vi "Apply Z scale to XY.vi"(6 "Enlarge Z scale?":bool, 8 "error in (no error)":errorcluster, 10 "Z Axis Ref":refnum<vi>, 11 "Plot Area Ref":refnum<vi>) -> (0 "error out":errorcluster)   [LabVIEW 2017, in "2D Compass.lvclass"]
uses:
  <vilib>/Math Plots/2D Math Plots/2D Compass/2D Compass/2D Compass.lvclass
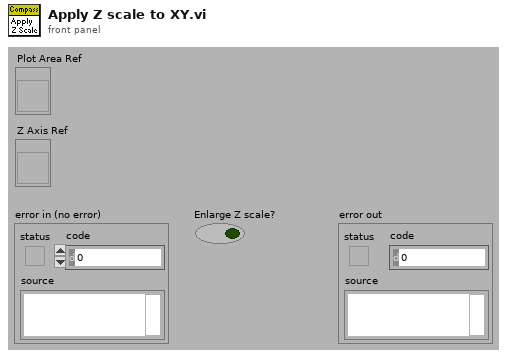
[diagram p1: front panel]
types:
  T1 = typedef "LVRectTypeDef.ctl" = cluster{"Left":i16, "Top":i16, "Right":i16, "Bottom":i16}
  T2 = typedef "LVPoint32TypeDef.ctl" = cluster{"Horizontal":i32, "Vertical":i32}
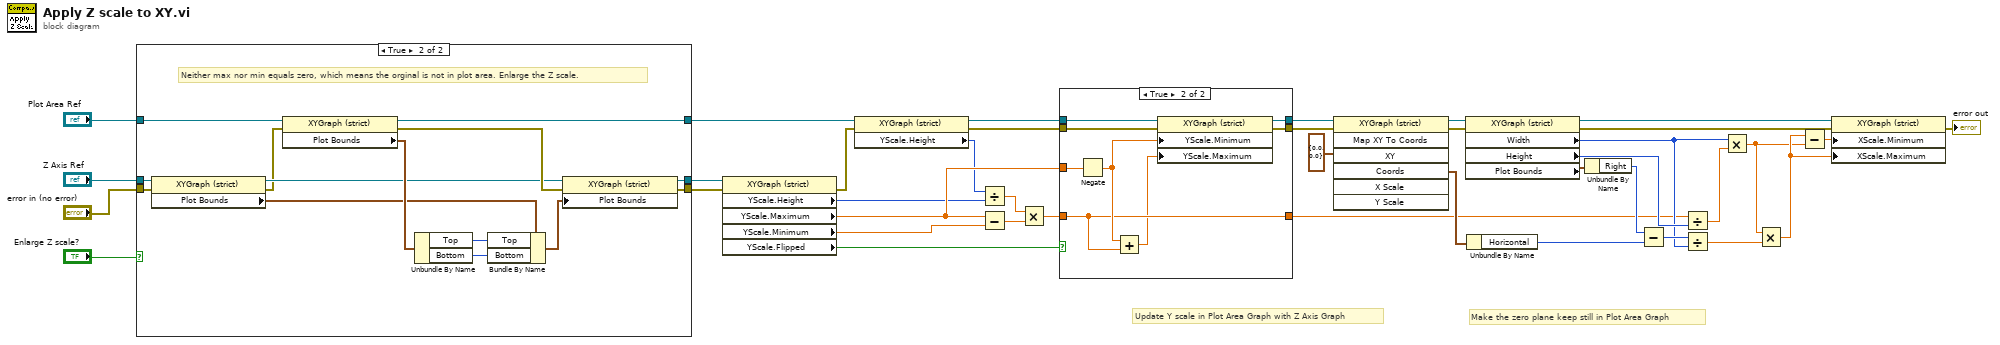
[diagram p0: block diagram]
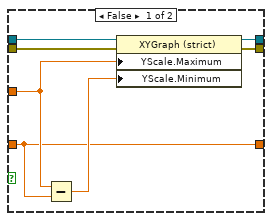
[diagram p3: hidden frame]
diagram:
  # "Make the zero plane keep still in Plot Area Graph"
  # "Update Y scale in Plot Area Graph with Z Axis Graph"
  n1 = case shown="True" "Enlarge Z scale?" {
    tunnel: [w40 w55] -> w6
    tunnel: "Plot Area Ref" -> [w40 w56]
    tunnel: [w42 w54] -> w4
    tunnel: "Z Axis Ref" -> [w42 w50]
    tunnel: [w41 w52] -> w2
    tunnel: "error in (no error)" -> [w41 w48]
    frame False {
    }
    frame True {
      # "Neither max nor min equals zero, which means the orginal is not in plot area. Enlarge the Z scale."
      n2 = property class="XYGraph (strict)"(reference=w50, error in=w48) -> (reference out=w49:refnum<vi>, error out=w47:errorcluster, "Plot Bounds"=w46:T1)
      n3 = property class="XYGraph (strict)"(reference=w56, error in=w47) -> (reference out=w55:refnum<vi>, error out=w53:errorcluster, "Plot Bounds"=w51:T1)
      n4 = Unbundle By Name(w51) -> ("Top"=w44:i16, "Bottom"=w43:i16)
      n5 = Bundle By Name(cluster=w46, "Top"=w44, "Bottom"=w43) -> (w45:T1)
      n6 = property class="XYGraph (strict)"(reference=w49, error in=w53, "Plot Bounds"=w45) -> (reference out=w54:refnum<vi>, error out=w52:errorcluster)
    }
  }
  n7 = property class="XYGraph (strict)"(reference=w4, error in=w2) -> (error out=w33:errorcluster, "YScale.Height"=w24:u32, "YScale.Maximum"=w32:dbl, "YScale.Minimum"=w31:dbl, "YScale.Flipped"=w30:bool)  [unwired: 1 out]
  n8 = property class="XYGraph (strict)"(reference=w6, error in=w33) -> (reference out=w26:refnum<vi>, error out=w34:errorcluster, "YScale.Height"=w25:u32)
  n9 = Divide(x=w25, y=w24) -> (x/y=w27:dbl)
  n10 = Subtract(x=w32, y=w31) -> (x-y=w28:dbl)
  n11 = Multiply(x=w27, y=w28) -> (x*y=w29:dbl)
  n12 = case shown="True" w30 {
    tunnel: w26 -> [w62 w70]
    tunnel: w29 -> [w58 w65]
    tunnel: w32 -> [w60 w67]
    tunnel: [w63 w71] -> w22
    tunnel: w34 -> [w61 w69]
    tunnel: [w58 w65] -> w9
    tunnel: [w57 w68] -> w23
    frame False {
      n13 = Subtract(x=w60, y=w58) -> (x-y=w59:dbl)
      n14 = property class="XYGraph (strict)"(reference=w62, error in=w61, "YScale.Maximum"=w60, "YScale.Minimum"=w59) -> (reference out=w57:refnum<vi>, error out=w63:errorcluster)
    }
    frame True {
      n15 = Negate(x=w67) -> (-x=w66:dbl)
      n16 = Add(x=w66, y=w65) -> (x+y=w64:dbl)
      n17 = property class="XYGraph (strict)"(reference=w70, error in=w69, "YScale.Minimum"=w66, "YScale.Maximum"=w64) -> (reference out=w68:refnum<vi>, error out=w71:errorcluster)
    }
  }
  n18 = invoke class="XYGraph (strict)" method="Map XY To Coords"(reference=w23, error in=w22, "XY"=cluster{"X":dbl, "Y":dbl} {"X"=0.0, "Y"=0.0}) -> (reference out=w20:refnum<vi>, error out=w21:errorcluster, "Coords"=w19:T2)  [unwired: 4 in, 4 out]
  n19 = property on="Property Node" class="XYGraph (strict)"(reference=w20, error in=w21) -> (reference out=w37:refnum<vi>, error out=w35:errorcluster, "Width"=w13:u32, "Height"=w38:u32, "Plot Bounds"=w17:T1)
  n20 = Unbundle By Name(w19) -> ("Horizontal"=w15:i32)
  n21 = Unbundle By Name(w17) -> ("Right"=w16:i16)
  n22 = Subtract(x=w16, y=w15) -> (x-y=w14:i32)
  n23 = Divide(x=w9, y=w38) -> (x/y=w12:dbl)
  n24 = Divide(x=w14, y=w13) -> (x/y=w11:dbl)
  n25 = Multiply(x=w13, y=w12) -> (x*y=w8:dbl)
  n26 = Multiply(x=w8, y=w11) -> (x*y=w10:dbl)
  n27 = Subtract(x=w10, y=w8) -> (x-y=w36:dbl)
  n28 = property on="Property Node" class="XYGraph (strict)"(reference=w37, error in=w35, "XScale.Minimum"=w36, "XScale.Maximum"=w10) -> (error out=→"error out":errorcluster)  [unwired: 1 out]
